vi "Load Settings from XML.vi"(8 "error in (no error)":errorcluster, 11 "Settings":T1) -> (0 "error out":errorcluster, 3 "Settings out":T1)   [LabVIEW 2019, in "Settings.lvlib"]
doc: "Attempts to load previous user specified settings from an XML file.\n\nThis VI will not generate an error. If a suitable XML file can't be loaded and parsed then it will simply return the default settings."
uses:
  Settings.lvlib
  Cluster - Settings.ctl
  MainController/Cluster - HardwareConfiguration.ctl
  MainController/Cluster - TestSettings.ctl
  <vilib>/Utility/xml.llb/Write to XML File(string).vi
  <vilib>/Utility/xml.llb/Read From XML File(string).vi
  MainController/MainController.lvlib
panel:
  # "(Scroll up for Settings Controls)"
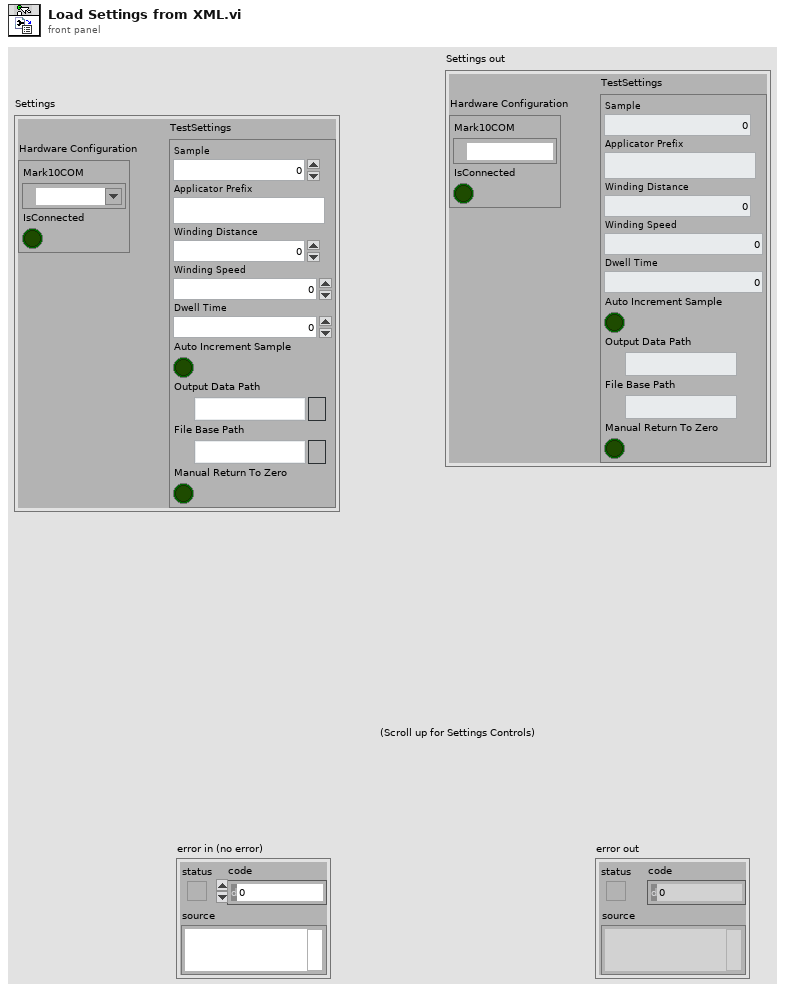
[diagram p1: front panel]
types:
  T1 = typedef "Settings.lvlib/Cluster - Settings.ctl" = cluster{"Hardware Configuration":T2, "TestSettings":T3}
  T2 = typedef "MainController.lvlib/Cluster - HardwareConfiguration.ctl" = cluster{"Mark10COM":refnum<visa-resource-name>, "IsConnected":bool}
  T3 = typedef "MainController.lvlib/Cluster - TestSettings.ctl" = cluster{"Sample":u32, "Applicator Prefix":string, "Winding Distance":dbl, "Winding Speed":dbl, "Dwell Time":dbl, "Auto Increment Sample":bool, "Output Data Path":path, "File Base Path":path, "Manual Return To Zero":bool}
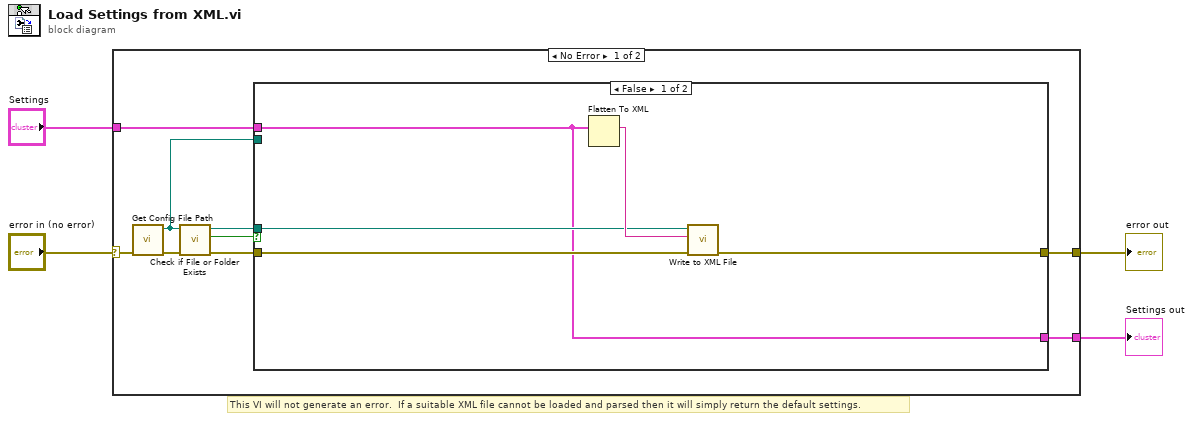
[diagram p0: block diagram]
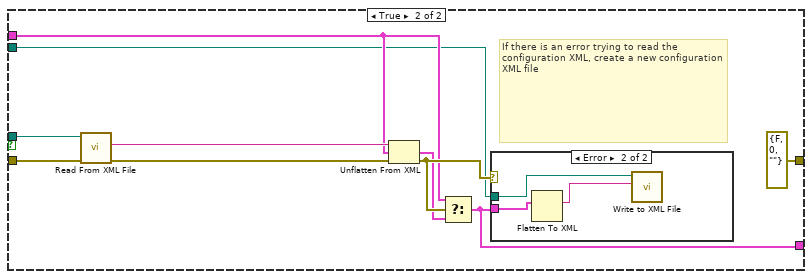
[diagram p2: hidden frame]
diagram:
  # "This VI will not generate an error.  If a suitable XML file cannot be loaded and parsed then it will simply return the default settings."
  n1 = case shown="No Error" "error in (no error)" {
    selector: "error in (no error)" -> [w12 w33]
    tunnel: [w5 w33] -> w3
    tunnel: "Settings" -> [w10 w32]
    tunnel: [w11 w32] -> w1
    frame No Error {
      n2 = call "Get Config File Path.vi"("error in (no error)"=w12) -> ("error out"=w13:errorcluster, "XML File Path"=w8:path)  [unwired: 9 in]
      n3 = call <vilib>:"Check if File or Folder Exists.vi"("error in (no error)"=w13, "path"=w8) -> ("error out"=w9:errorcluster, "file or folder exists?"=w6:bool, "dup path"=w7:path)  [unwired: 7 in]
      n4 = case shown="False" w6 {
        tunnel: [w14 w27] -> w11
        tunnel: w10 -> [w14 w24]
        tunnel: w9 -> [w17 w22]
        tunnel: w8 -> [_ w21]
        tunnel: w7 -> [w16 w20]
        tunnel: [w15 errorcluster {"status"=FALSE, "code"=0, "source"=""} ("error out")] -> w5
        frame False {
          n5 = Flatten To XML(anything=w14) -> (xml string=w18:string)
          n6 = call-poly <vilib>:"Write to XML File.vi"("error in (no error)"=w17, "XML Input"=w18, "XML File Path"=w16) -> ("error out"=w15:errorcluster)  [unwired: 6 in, 2 out]
        }
        frame True {
          # "If there is an error trying to read the configuration XML, create a new configuration XML file"
          n7 = call-poly <vilib>:"Read From XML File.vi"("error in (no error)"=w22, "XML File Path"=w20) -> ("error out"=w26:errorcluster, "XML Elements"=w28:string)  [unwired: 7 in, 1 out]
          n8 = Unflatten From XML(xml string=w28, type=w24, error in (no error)=w26) -> (value=w23:T1, error out=w25:errorcluster)
          n9 = Select(t=w24, s=w25, f=w23) -> (s? t:f=w27:T1)
          n10 = case shown="Error" w25 {
            tunnel: w27 -> [_ w31]
            tunnel: w21 -> [_ w29]
            frame No Error {
            }
            frame Error {
              n11 = Flatten To XML(anything=w31) -> (xml string=w30:string)
              n12 = call-poly <vilib>:"Write to XML File.vi"("XML Input"=w30, "XML File Path"=w29) -> ()  [unwired: 7 in, 3 out]
            }
          }
        }
      }
    }
    frame Error {
    }
  }
  "error out" <- w3
  "Settings out" <- w1
